vi "PathFunctions_CreateFolderStructureRecoursively.vi"(0 "Path":path, 5 "ErrorIn":errorcluster) -> (14 "Path(dup)":path, 16 "CreatedNewFolder(s)":bool, 19 "ErrorOut":errorcluster)   [LabVIEW 2016]
doc: "Erzeugt eine rekursive Ordnerstruktur\n\n15.04.14 / sige"
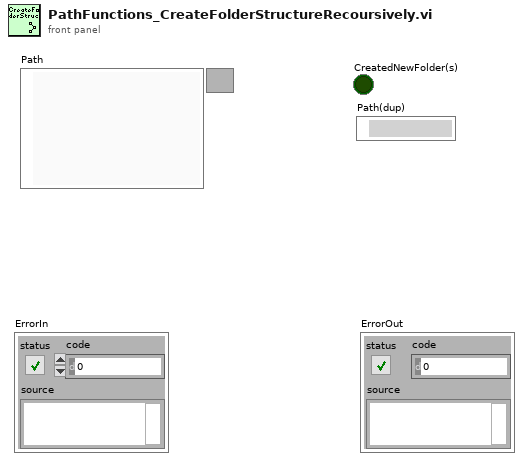
[diagram p1: front panel]
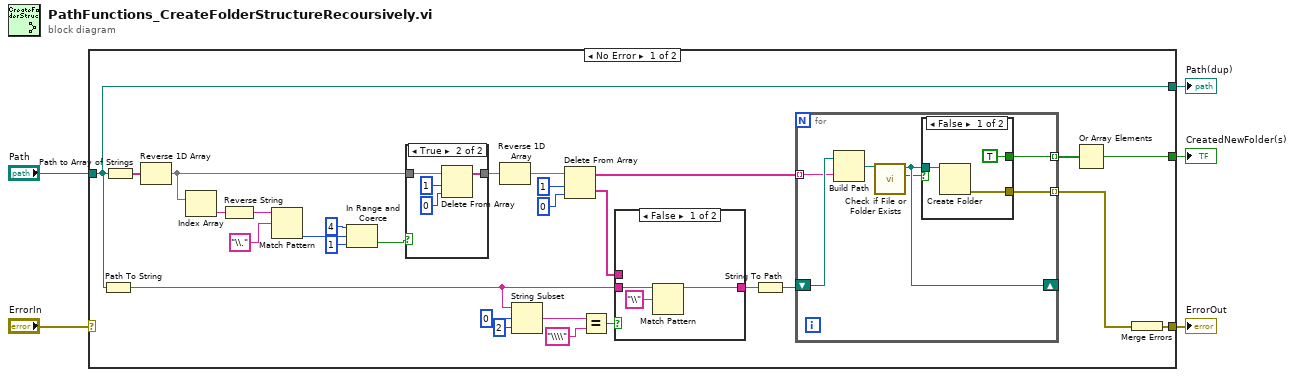
[diagram p0: block diagram]
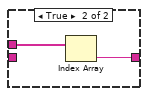
[diagram p2: hidden frame]
diagram:
  n1 = case shown="No Error" "ErrorIn" {
    selector: "ErrorIn" -> [_ w55]
    tunnel: [w20 w55] -> w4
    tunnel: "Path" -> [w17 w54]
    tunnel: [w18 _] -> w2
    tunnel: [w17 w54] -> w1
    frame No Error {
      n2 = Path To String(path=w17) -> (string=w12:string)
      n3 = Path to Array of Strings(0:w17) -> (2:w25:string[])  [unwired: 1 out]
      n4 = Reverse 1D Array(array=w25) -> (reversed array=w26:string[])
      n5 = Index Array(array=w26) -> (element=w29:string)  [unwired: 1 in]
      n6 = Reverse String(1:w29) -> (0:w28:string)
      n7 = Match Pattern(string=w28, regular expression="\\.") -> (offset past match=w16:i32)  [unwired: 1 in, 3 out]
      n8 = In Range and Coerce(upper limit=4, x=w16, lower limit=1) -> (In Range?=w13:bool)  [unwired: 1 out]
      n9 = case shown="True" w13 {
        tunnel: w26 -> [w39 w43]
        tunnel: [w39 w40] -> w24
        frame False {
        }
        frame True {
          n10 = Delete From Array(array=w43, length=1, index=0) -> (array with subset deleted=w40:string[])  [unwired: 1 out]
        }
      }
      n11 = Reverse 1D Array(array=w24) -> (reversed array=w23:string[])
      n12 = String Subset(string=w12, offset (0)=0, length (rest)=2 ("length (rest)")) -> (substring=w9:string)
      n13 = Delete From Array(array=w23, length=1, index=0) -> (deleted portion=w6:string[], array with subset deleted=w30:string[])
      n14 = Equal?(x=w9, y="\\\\") -> (x = y?=w7:bool)
      n15 = case shown="False" w7 {
        tunnel: [w35 w37] -> w22
        tunnel: w12 -> [w34 _]
        tunnel: w6 -> [_ w38]
        frame False {
          n16 = Match Pattern(string=w34, regular expression="\\") -> (before substring=w35:string)  [unwired: 1 in, 3 out]
        }
        frame True {
          n17 = Index Array(array=w38) -> (element=w37:string)  [unwired: 1 in]
        }
      }
      n18 = String To Path(string=w22) -> (path=w31:path)
      n19 = for {
        tunnel: w30 -> [w49] mode=indexing
        shift-right: [w46] -> _
        shift-left: w31 -> [w50]
        tunnel: [w47] -> w21 mode=indexing
        tunnel: [w44] -> w19 mode=indexing
        n20 = Build Path(base path=w50, name or relative path=w49) -> (appended path=w48:path)
        n21 = call <vilib>:"Check if File or Folder Exists.vi"("path"=w48) -> ("file or folder exists?"=w45:bool, "dup path"=w46:path)  [unwired: 8 in, 1 out]
        n22 = case shown="False" w45 {
          tunnel: w46 -> [w53 _]
          tunnel: [w52 _] -> w47
          tunnel: [TRUE _] -> w44
          frame False {
            n23 = Create Folder(path (use dialog)=w53) -> (error out=w52:errorcluster)  [unwired: 2 in, 2 out]
          }
          frame True {
          }
        }
      }
      n24 = Or Array Elements(Boolean array=w19) -> (logical OR=w18:bool)
      n25 = Merge Errors(w21) -> (w20:errorcluster)
    }
    frame Error {
    }
  }
  "ErrorOut" <- w4
  "CreatedNewFolder(s)" <- w2
  "Path(dup)" <- w1
